vi "AutoHelper_DelayedAction.vi"(6 "Pass_Through_Time":dbl=-1.0 format="%33.4f", 9 "Delay Time Sec":dbl, 11 "New Step":bool) -> (0 "Timeout ALT":bool, 1 "Remaining Delay Time Sec":dbl, 2 "Delayed Action Pulse":bool, 3 "Delayed Action":bool, 4 "Remaining ALT":dbl)   [LabVIEW 2019, in "Trajectory_Library.lvlib"]
doc: "Implements a simplified state machine similar to a mechanical / electrical drum sequencer. When the Drum Sequencer is \"Ready\" and the \"Initiate\" input becomes TRUE,, the drum sequences through its set of steps from 1 to N. After each Step is executed it is followed by a wait. During the wait the Step output indicates \"Do Nothing\". The number of Steps is determined by the number of elements in the \"Step Times\" input array. Once all the steps have been executed, the Drum Sequencer cycles bac to wait for another initiate. \n\nThere is a Cancel input that interrupts the sequence, executes the Cancel Step, performs the cancel wait, and then returns to wait for an Initiate action. \n\nIf any of the Step Times, or Cancel times are negative, or there more than 32 steps, or less than 1 step an error is signaled. The drum sequencer selects the error state and stays there.\n\nInputs:\n\nOutputs:"
uses:
  Trajectory_Library.lvlib
  Util_GetTime_U32.vi
  Util_GetTime_U64.vi
  <vilib>/Utility/semaphor.llb/Obtain Semaphore Reference.vi
  Timer_Reset.vi
  Timer_Start.vi
  Timer_Stop.vi
panel:
  # "For Debug"
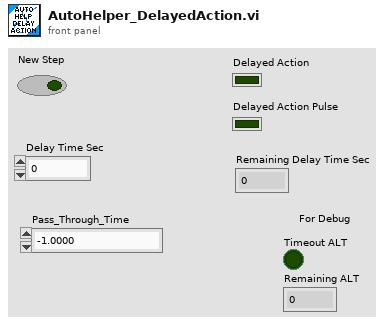
[diagram p1: front panel]
types:
  T1 = typedef "Trajectory_Library.lvlib/TIMER.ctl" = cluster{"StartTime":dbl, "Accumulated TIme":dbl, "Running":bool, "semaphore":T2}
  T2 = typedef "Semaphore RefNum" = refnum<k1>
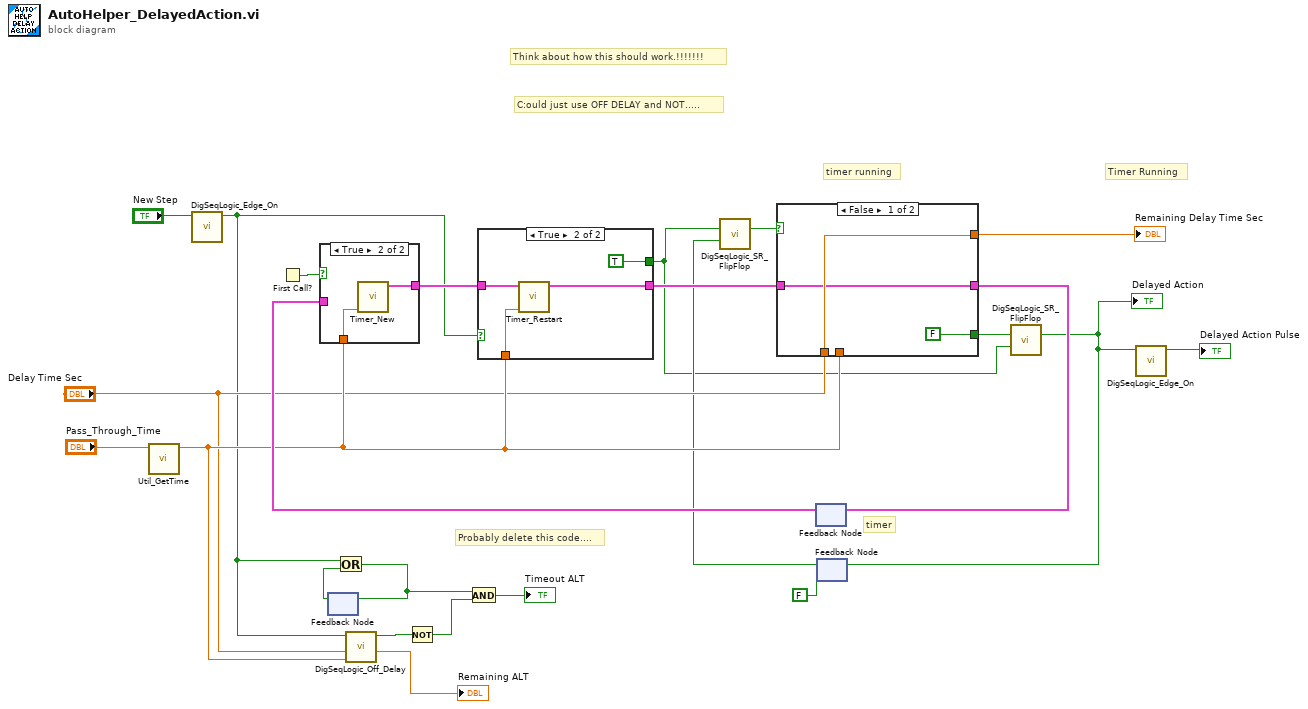
[diagram p0: block diagram]
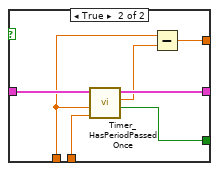
[diagram p2: hidden frame]
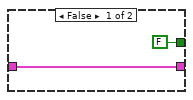
[diagram p3: hidden frame]
diagram:
  # "Probably delete this code...."
  # "Think about how this should work.!!!!!!!"
  # "C:ould just use OFF DELAY and NOT....."
  # "timer running"
  # "Timer Running"
  # "timer"
  n1 = call "Util_GetTime.vi"("Pass_Through_Time"="Pass_Through_Time") -> ("FPGA_Time_Seconds"=w14:dbl)  [unwired: 8 in, 2 out]
  n2 = call "DigSeqLogic_Edge_On.vi"("Input"="New Step") -> ("On Edge"=w9:bool)  [unwired: 10 in]
  n3 = First Call?() -> (First Call?: T/F=w22:bool)
  n4 = feedback #1() -> (w10:bool)  [unwired: 1 in]
  n5 = Or(x=w9, y=w10) -> (x .or. y?=w6:bool)
  n6 = feedback-in #1(w6) -> ()
  n7 = call "DigSeqLogic_Off_Delay.vi"("Time"=w14, "Delay"="Delay Time Sec", "Input"=w9) -> ("Remain"=→"Remaining ALT":dbl, "Output"=w12:bool)  [unwired: 7 in]
  n8 = Not(x=w12) -> (.not. x?=w8:bool)
  n9 = And(x=w6, y=w8) -> (x .and. y?=→"Timeout ALT":bool)
  n10 = feedback #2() -> (w21:T1)  [unwired: 1 in]
  n11 = case shown="True" w22 {
    tunnel: [w25 w27] -> w20
    tunnel: w14 -> [_ w26]
    tunnel: w21 -> [w25 _]
    frame False {
    }
    frame True {
      n12 = call "Timer_New.vi"("Pass_Through_Time"=w26) -> ("TIMER"=w27:T1)  [unwired: 10 in]
    }
  }
  n13 = case shown="True" w9 {
    tunnel: [w29 w33] -> w19
    tunnel: w20 -> [w29 w32]
    tunnel: w14 -> [_ w31]
    tunnel: [FALSE TRUE] -> w3
    frame False {
    }
    frame True {
      n14 = call "Timer_Restart.vi"("Pass_Through_Time"=w31, "in Timer"=w32) -> ("out Timer"=w33:T1)  [unwired: 9 in]
    }
  }
  n15 = feedback #3(FALSE ("Expired")) -> (w5:bool)
  n16 = call "DigSeqLogic_SR_FlipFlop.vi"("Set"=w3, "Reset"=w5) -> ("Output"=w16:bool)  [unwired: 12 in, 1 out]
  n17 = case shown="False" w16 {
    tunnel: w19 -> [w35 w43]
    tunnel: w14 -> [_ w42]
    tunnel: [w35 w41] -> w18
    tunnel: "Delay Time Sec" -> [w36 w40]
    tunnel: [w36 w38] -> w17
    tunnel: [FALSE ("Expired") w37] -> w4
    frame False {
    }
    frame True {
      n18 = call "Timer_HasPeriodPassedOnce.vi"("Pass_Through_Time"=w42, "Period"=w40, "in Timer"=w43) -> ("Expired"=w37:bool, "CurrentTImer"=w39:dbl, "out Timer"=w41:T1)  [unwired: 6 in]
      n19 = Subtract(x=w40, y=w39) -> (x-y=w38:dbl)
    }
  }
  "Remaining Delay Time Sec" <- w17
  n20 = feedback-in #2(w18) -> ()
  n21 = call "DigSeqLogic_SR_FlipFlop.vi"("Set"=w4, "Reset"=w3) -> ("Output"=w2:bool)  [unwired: 12 in, 1 out]
  "Delayed Action" <- w2
  n22 = feedback-in #3(w2) -> ()
  n23 = call "DigSeqLogic_Edge_On.vi"("Input"=w2) -> ("On Edge"=→"Delayed Action Pulse":bool)  [unwired: 10 in]
